vi "Find Interval.vi"(8 "error in (no error)":errorcluster, 11 "UI Data":T1) -> (0 "error out":errorcluster, 3 "Interval":T3)   [LabVIEW 2026]
uses:
  controls/Schedule Interval.ctl
  controls/UI Data.ctl
  controls/User Settings.ctl
  controls/System Status Displays.ctl
  controls/Manual Override.ctl
  controls/Global Settings.ctl
panel:
  in  "Minutes":i32
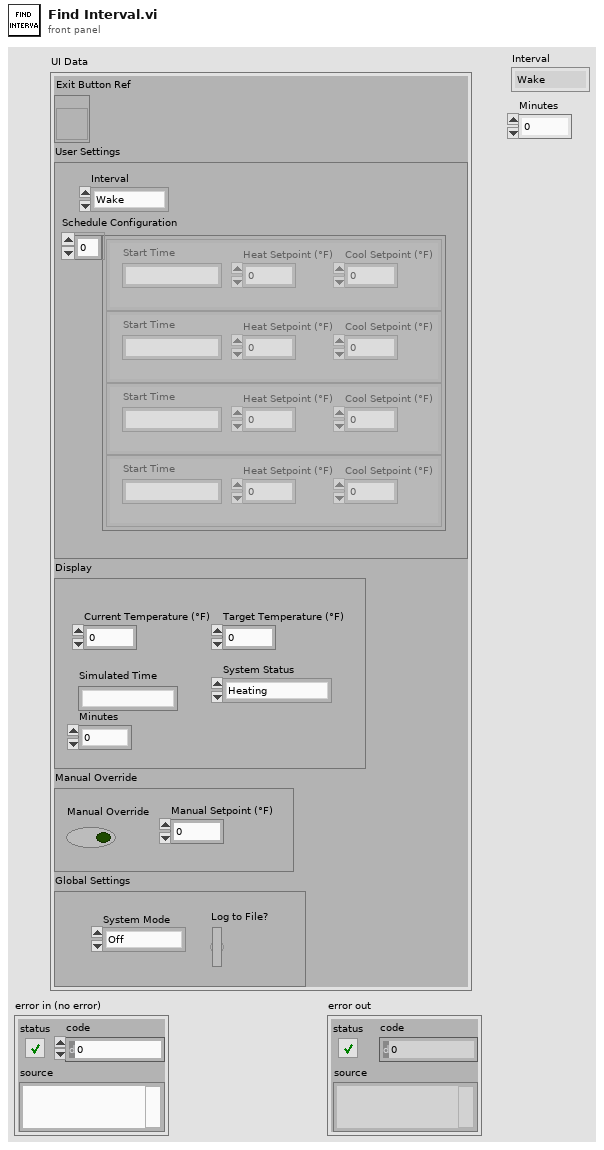
[diagram p1: front panel]
types:
  T1 = typedef "UI Data.ctl" = cluster{"Exit Button Ref":refnum<vi>, "User Settings":T2, "Display":T4, "Manual Override":T5, "Global Settings":T6}
  T2 = typedef "User Settings.ctl" = cluster{"Schedule Configuration":cluster{"Start Time":string, "Heat Setpoint (°F)":dbl, "Cool Setpoint (°F)":dbl}[], "Interval":T3}
  T3 = typedef "Schedule Interval.ctl" = enum16{"Wake", "Leave", "Return", "Sleep"}
  T4 = typedef "System Status Displays.ctl" = cluster{"Current Temperature (°F)":dbl, "Target Temperature (°F)":dbl, "System Status":enum16{"Heating", "Cooling", "Idle"}, "Simulated Time":string, "Minutes":i16}
  T5 = typedef "Manual Override.ctl" = cluster{"Manual Override":bool, "Manual Setpoint (°F)":dbl}
  T6 = typedef "Global Settings.ctl" = cluster{"System Mode":enum16{"Off", "Cool", "Auto", "Heat"}, "Log to File?":bool}
  T7 = cluster{"Start Time":string, "Heat Setpoint (°F)":dbl, "Cool Setpoint (°F)":dbl}[]
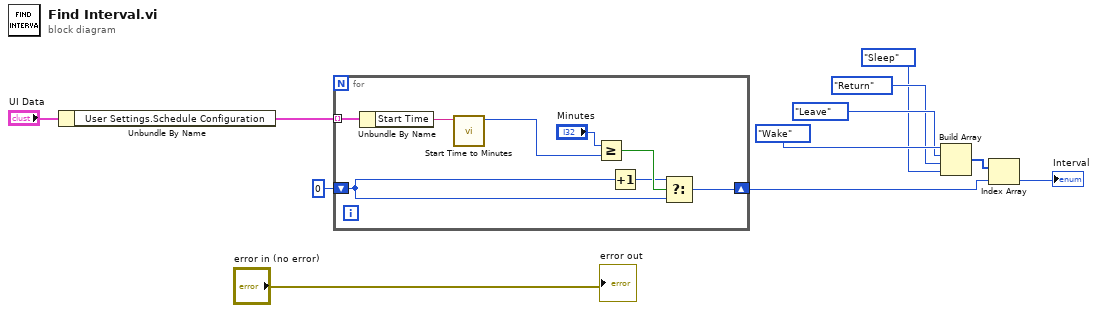
[diagram p0: block diagram]
diagram:
  n1 = Unbundle By Name("UI Data") -> ("User Settings.Schedule Configuration"=w9:T7)
  n2 = for {
    tunnel: w9 -> [w19] mode=indexing
    shift-right: [w14] -> w1
    shift-left: 0 -> [w12]
    n3 = Unbundle By Name(w19) -> ("Start Time"=w18:string)
    n4 = call "Start Time to Minutes.vi"("Start Time"=w18) -> ("Minutes"=w16:i32)  [unwired: 9 in, 1 out]
    n5 = Greater Or Equal?(x="Minutes", y=w16) -> (x >= y?=w15:bool)
    n6 = Increment(x=w12) -> (x+1=w13:i32)
    n7 = Select(t=w13, s=w15, f=w12) -> (s? t:f=w14:i32)
  }
  n8 = Build Array(Schedule_Interval."Wake", Schedule_Interval."Leave", Schedule_Interval."Return", Schedule_Interval."Sleep") -> (w4:T3[])
  n9 = Index Array(array=w4, index=w1) -> (element=→"Interval":T3)
  "error out" <- "error in (no error)"
